vi "Write Scrubber.vi"(8 "error in":errorcluster, 10 "Scrubber":refnum<class "Scrubber.lvclass">, 11 "Options in":refnum<class "Options.lvclass">) -> (0 "error out":errorcluster, 3 "Options out":refnum<class "Options.lvclass">)   [LabVIEW 2020, in "Approval Tests.lvlib" / "Options.lvclass"]
uses:
  Options.lvclass
  Scrubber/Scrubber.lvclass
  Options.lvclass/Options.ctl
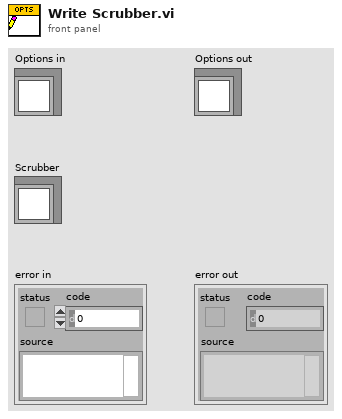
[diagram p1: front panel]
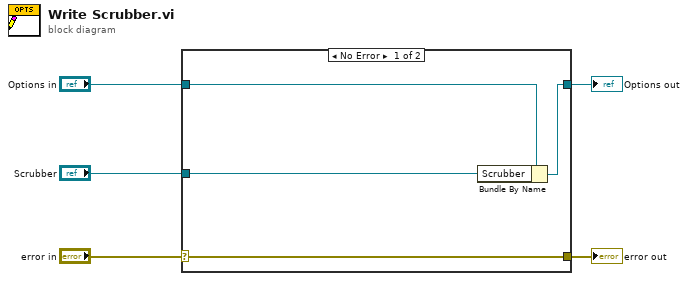
[diagram p0: block diagram]
diagram:
  n1 = case shown="No Error" "error in" {
    selector: "error in" -> [w9 w11]
    tunnel: [w9 w11] -> w4
    tunnel: [w7 w10] -> w2
    tunnel: "Options in" -> [w8 w10]
    tunnel: "Scrubber" -> [w6 _]
    frame No Error {
      n2 = Bundle By Name(cluster=w8, "Scrubber"=w6) -> (w7:refnum<class "Options.lvclass">)
    }
    frame Error {
    }
  }
  "error out" <- w4
  "Options out" <- w2
